vi "Global Value_charles.vi"() -> ()   [LabVIEW 2011, in "Lock-In Variable Channels_2.lvclass"]
uses:
  Variable Channel O.O.P/Lock-In Variable Channels_2.lvclass
panel:
  in  "Channel Setting 2":T1(array[cluster])=[{"Channel"=1, "Gain"=1, "Shunt Resistor"=5, "Measure"=1}, {"Channel"=2, "Gain"=1, "Shunt Resistor"=5, "Measure"=1}, {"Channel"=3, "Gain"=1, "Shunt Resistor"=1, "Measure"=2}, {"Channel"=4, "Gain"=1, "Shunt Resistor"=1, "Measure"=2}] {"Measure" items=["Float", "Current(Diff)", "Voltage(SE+)"]; "Shunt Resistor" items=["Open"=1, "50 Ohms"=2, "500 Ohms"=3, "5k Ohms"=4, "50k Ohms"=5]; "Gain" items=["1x"=1, "10x"=2, "100x"=3, "1000x"=4]; "Channel" items=["Channel 1"=1, "Channel 2"=2, "Channel 3"=3, "Channel 4"=4, "Channel 5"=5, "Channel 6"=6, "Channel 7"=7, "Channel 8"=8]}
  out "Lock-in results":dbl[][](array[numeric])=[[-2.517270477296176e-06, 7.334704760705008e-09, 2.5172811630330144e-06, 0.0035966610942982525], [2.5054303804978227e-06, -8.295456619278016e-09, 2.505444113549929e-06, -3.7941019658616143e-06], [0.37442750320093354, -0.0011972063596659593, 0.37442941718881106, -0.18319871608958335], [0.12520740572879255, -0.00040862747457553973, 0.12520807252628502, -0.18699010994582346]]
  out "Reset Lockin":bool
  out "Stop Lockin":bool
  in  "Channel Setting":T2(array[cluster])=[{"Channel"=1, "Gain"=1, "Shunt Resistor"=5, "Measure"=1, "Output"={"Signal Type"=enum."Triangle Wave", "frequency"=0.25, "Amplitude"=1.0, "Phase"=0.0, "DC"=0.0}}, {"Channel"=2, "Gain"=1, "Shunt Resistor"=5, "Measure"=1, "Output"={"Signal Type"=enum."Triangle Wave", "frequency"=0.25, "Amplitude"=0.0, "Phase"=0.0, "DC"=0.0}}, {"Channel"=3, "Gain"=1, "Shunt Resistor"=1, "Measure"=2, "Output"={"Signal Type"=enum."Triangle Wave", "frequency"=0.25, "Amplitude"=0.0, "Phase"=0.0, "DC"=0.0}}, {"Channel"=4, "Gain"=1, "Shunt Resistor"=1, "Measure"=2, "Output"={"Signal Type"=enum."Triangle Wave", "frequency"=0.25, "Amplitude"=0.0, "Phase"=0.0, "DC"=0.0}}] {"Output"."DC" format="%.2p"; "Output"."frequency" format="%0.2p"; "Measure" items=["Float", "Current", "Voltage"]; "Shunt Resistor" items=["Open"=1, "50 Ohms"=2, "500 Ohms"=3, "5k Ohms"=4, "50k Ohms"=5]; "Gain" items=["1x"=1, "10x"=2, "100x"=3, "1000x"=4]; "Channel" items=["Channel 1"=1, "Channel 2"=2, "Channel 3"=3, "Channel 4"=4, "Channel 5"=5, "Channel 6"=6, "Channel 7"=7, "Channel 8"=8]}
  in  "iteration":i8
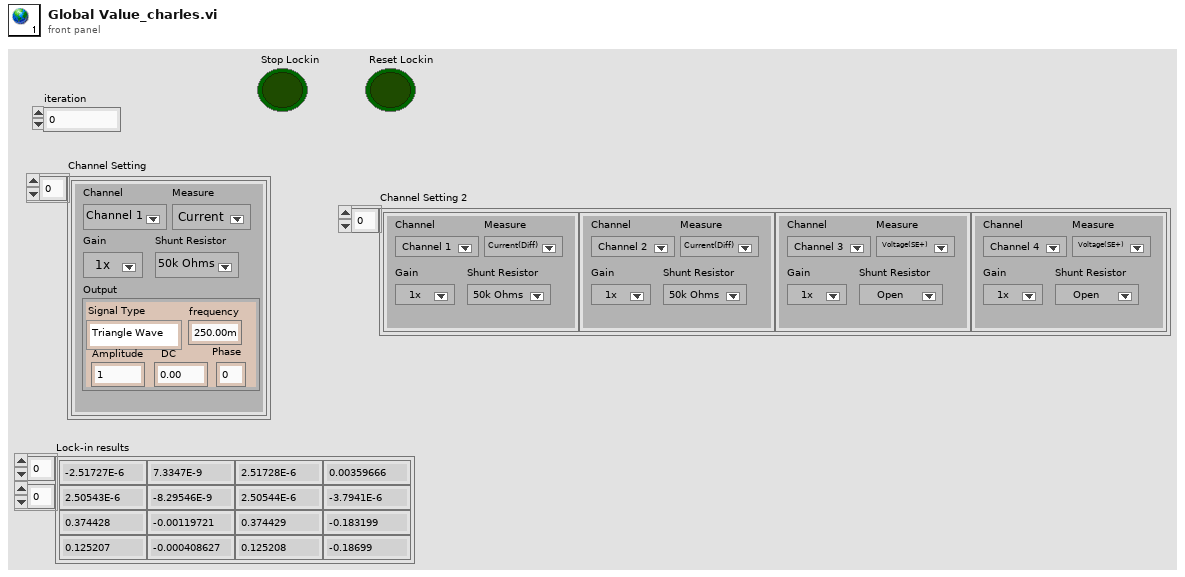
[diagram p1: front panel]
types:
  T1 = cluster{"Channel":u16, "Gain":u16, "Shunt Resistor":u16, "Measure":u16}[]
  T2 = cluster{"Channel":u16, "Gain":u16, "Shunt Resistor":u16, "Measure":u16, "Output":cluster{"Signal Type":enum16{"Sine Wave", "Triangle Wave", "Square Wave", "Sawtooth Wave"}, "frequency":dbl, "Amplitude":dbl, "Phase":dbl, "DC":dbl}}[]
diagram:
